vi "2 update_mission_queue_TEST.vi"() -> ()   [LabVIEW 2011]
uses:
  2 Typedefs/UTM Location.ctl
  2 Classes/Mission/Mission.lvclass
  2 Classes/MissionQueue/MissionQueue.lvclass
panel:
  in  "Point of Interest 4":T1 {"North" format="%#_10f"; "East" format="%#_8f"}
  in  "Point of Interest 3":T1 {"North" format="%#_10f"; "East" format="%#_8f"}
  in  "Point of Interest 2":T1 {"North" format="%#_10f"; "East" format="%#_8f"}
  in  "Point of Interest":T1 {"North" format="%#_10f"; "East" format="%#_8f"}
  in  "Mission Type":T2(ring)
  # "PoI order for stationkeeping:\nNW, NE, SW, SE"
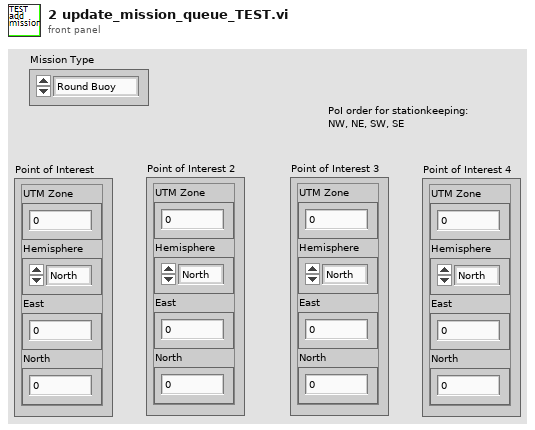
[diagram p1: front panel]
types:
  T1 = typedef "UTM Location.ctl" = cluster{"UTM Zone":dbl, "Hemisphere":enum16{"North", "South"}, "East":dbl, "North":dbl}
  T2 = enum16{"Round Buoy", "Pass Buoys", "Station Keeping"}
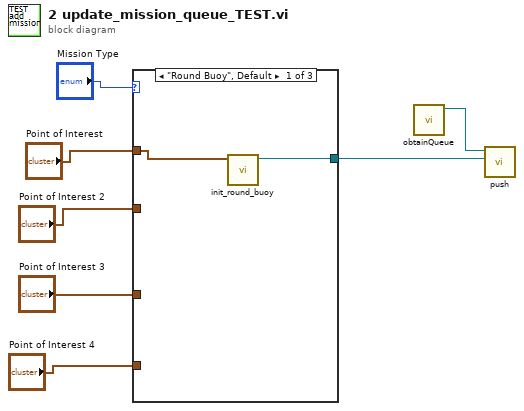
[diagram p0: block diagram]
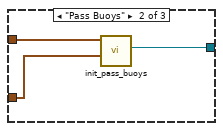
[diagram p2: hidden frame]
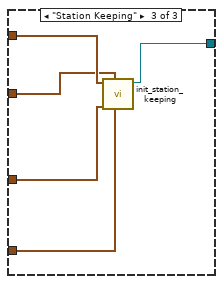
[diagram p3: hidden frame]
diagram:
  n1 = case shown="\"Round Buoy\", Default" "Mission Type" {
    tunnel: "Point of Interest" -> [w9 w12 w17]
    tunnel: "Point of Interest 2" -> [_ w11 w16]
    tunnel: "Point of Interest 4" -> [_ _ w14]
    tunnel: "Point of Interest 3" -> [_ _ w15]
    tunnel: [w8 w10 w13] -> w1
    frame "Round Buoy", Default {
      n2 = call "init_round_buoy.vi"("Buoy to Round"=w9) -> ("Mission out"=w8:refnum<class "Mission.lvclass">)  [unwired: 10 in]
    }
    frame "Pass Buoys" {
      n3 = call "init_pass_buoys.vi"("Buoy Pass 2"=w11, "Buoy Pass 1"=w12) -> ("Mission.lvclass"=w10:refnum<class "Mission.lvclass">)  [unwired: 9 in]
    }
    frame "Station Keeping" {
      n4 = call "init_station_keeping.vi"("Buoy SE"=w14, "Buoy NE"=w16, "Buoy SW"=w15, "Buoy NW"=w17) -> ("Mission out"=w13:refnum<class "Mission.lvclass">)  [unwired: 7 in]
    }
  }
  n5 = call "obtainQueue.vi"() -> ("MissionQueue.lvclass"=w2:refnum<class "MissionQueue.lvclass">)  [unwired: 10 in, 1 out]
  n6 = call "push.vi"("Mission.lvclass"=w1, "MissionQueue in"=w2) -> ()  [unwired: 8 in, 2 out]
